vi "Init Wrist.vi"() -> (3 "Wrist Out":T2={"DeviceStatus"={"status"=FALSE, "code"=0, "source"=""}, "Type"=enum."CAN", "PWM"={"PWM Channel"=enum."PWM 1", "DeadBand"={"Name"="", "maxPositivePwm"=0, "minPositivePwm"=0, "centerPwm"=0, "maxNegativePwm"=0, "minNegativePwm"=0, "angularRange"=0}}, "CAN"={"Device Number"=1, "SetOutput VI Ref"=variant(refnum<vi> refnum), "GetOutput VI Ref"=variant(refnum<vi> refnum), "Enable VI Ref"=variant(refnum<vi> refnum), "Disable VI Ref"=variant(refnum<vi> refnum), "Data"=variant(cluster{"Library":path, "handle":u64, "Control Mode":u16, "UsageFrame":u32, "RefNumName":string, "arbID":u32} {"Library"=path "libCTRE_PhoenixCCI.so", "handle"=2992853744, "Control Mode"=0, "UsageFrame"=0, "RefNumName"="Wrist", "arbID"=33816577})}, "Invert"=FALSE, "DIO PWM"={"PWM \"Enable\" Channel"=enum."Invalid", "DIOChannel"=enum."Invalid", "PWM Rate"=0.0}})   [LabVIEW 2018]
uses:
  <vilib>/Rock Robotics/WPI/MotorControl/WPI_MotorControlDeviceRef.ctl
  <vilib>/Rock Robotics/WPI/MotorControl/WPI_MotorControlType.ctl
  <vilib>/Rock Robotics/SystemInterfaces/DIO/FPGA_DIOPWMChannel.ctl
  <vilib>/Rock Robotics/WPI/PWM/WPI_PWMDeadband.ctl
  <vilib>/Rock Robotics/SystemInterfaces/DIO/FPGA_DIOChannel.ctl
  <vilib>/Rock Robotics/WPI/ThirdParty/Phoenix-LabVIEW/Motor Controller/Controls/CTRE_Phoenix_MotorControl_NeutralMode.ctl
  <vilib>/Rock Robotics/WPI/ThirdParty/Phoenix-LabVIEW/Motor Controller/Controls/CTRE_Phoenix_MotorControl_FeedbackDevice.ctl
panel:
  in  "Deadband":dbl
  in  "Max Velocity":i32=1000
  in  "Max Accel":i32=1000
  in  "PID Constants":T1={"P Gain"=1.0, "I Gain"=0.002, "D Gain"=0.1, "F Gain"=0.0, "I Zone"=300.0, "Min Output"=-1.0, "Max Output"=1.0}
  in  "Enable Current Limit?":bool=TRUE
  in  "Peak Current Maximum Duration (ms)":i32
  in  "Peak Current (Amps)":i32
  in  "Continuous Current Limit (Amps)":i32=30
  in  "Invert":bool=TRUE
  in  "Sensor Inverted":bool=TRUE
  in  "Device Number":u8=5
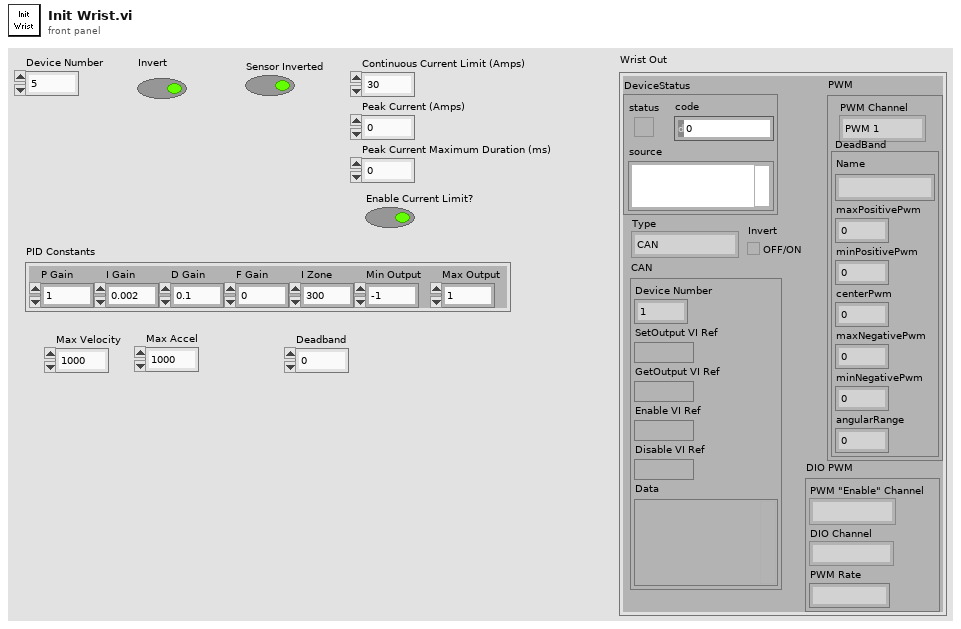
[diagram p1: front panel]
types:
  T1 = cluster{"P Gain":dbl, "I Gain":dbl, "D Gain":dbl, "F Gain":dbl, "I Zone":dbl, "Min Output":dbl, "Max Output":dbl}
  T2 = typedef "WPI_MotorControlDeviceRef.ctl" = cluster{"DeviceStatus":errorcluster, "Type":T3, "PWM":cluster{"PWM Channel":T4, "DeadBand":T5}, "CAN":cluster{"Device Number":u8, "SetOutput VI Ref":variant, "GetOutput VI Ref":variant, "Enable VI Ref":variant, "Disable VI Ref":variant, "Data":variant}, "Invert":bool, "DIO PWM":cluster{"PWM \"Enable\" Channel":T4, "DIOChannel":T6, "PWM Rate":dbl}}
  T3 = typedef "WPI_MotorControlType.ctl" = enum16{"PWM", "CAN", "DIO PWM"}
  T4 = typedef "FPGA_DIOPWMChannel.ctl" = enum8{"PWM 0", "PWM 1", "PWM 2", "PWM 3", "PWM 4", "PWM 5", "PWM 6", "PWM 7", "PWM 8", "PWM 9", "PWM MXP 0", "PWM MXP 1", "PWM MXP 2", "PWM MXP 3", "PWM MXP 4", "PWM MXP 5", "PWM MXP 6", "PWM MXP 7", "PWM MXP 8", "PWM MXP 9", "Invalid"}
  T5 = typedef "WPI_PWMDeadband.ctl" = cluster{"Name":string, "maxPositivePwm":i32, "minPositivePwm":i32, "centerPwm":i32, "maxNegativePwm":i32, "minNegativePwm":i32, "angularRange":u16}
  T6 = typedef "FPGA_DIOChannel.ctl" = enum8{"DIO 0", "DIO 1", "DIO 2", "DIO 3", "DIO 4", "DIO 5", "DIO 6", "DIO 7", "DIO 8", "DIO 9", "DIO MXP 0", "DIO MXP 1", "DIO MXP 2", "DIO MXP 3", "DIO MXP 4", "DIO MXP 5", "DIO MXP 6", "DIO MXP 7", "DIO MXP 8", "DIO MXP 9", "DIO MXP 10", "DIO MXP 11", "DIO MXP 12", "DIO MXP 13", "DIO MXP 14", "DIO MXP 15", "SPI Port CS1", "SPI Port CS2", "SPI Port CS3", "SPI Port MISO", "SPI Port MOSI", "Invalid"}
  T7 = typedef "CTRE_Phoenix_MotorControl_FeedbackDevice.ctl" = i8
  T8 = typedef "CTRE_Phoenix_MotorControl_NeutralMode.ctl" = enum8{"EEPROMSetting", "Override to Coast", "Override to Brake"}
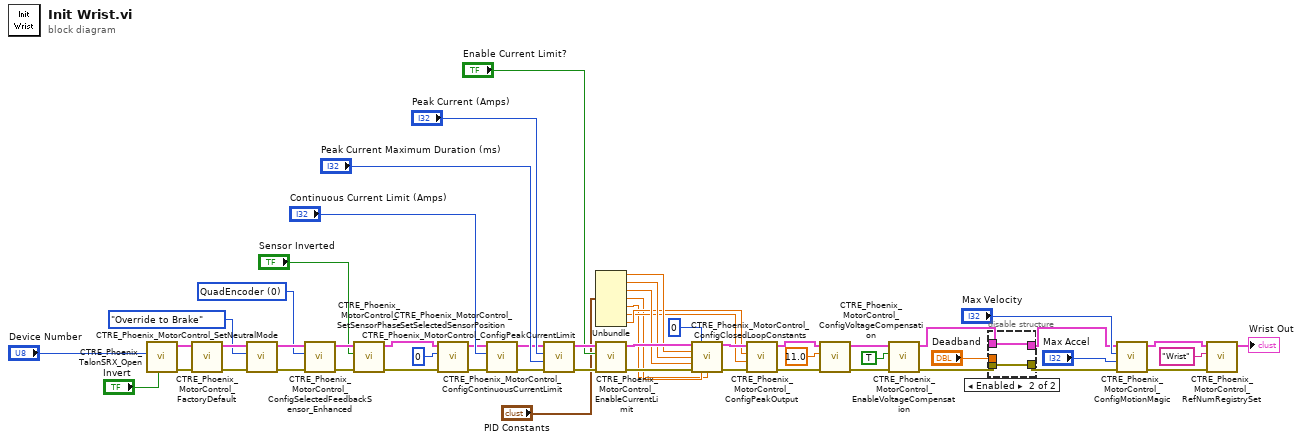
[diagram p0: block diagram]
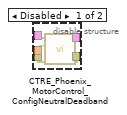
[diagram p2: hidden frame]
diagram:
  w47 = T7 0 items=["QuadEncoder"=0, "Analog"=2, "Tachometer"=4, "Pulse Width Encoded Position"=8, "Sensor Sum (S0 + S1)"=9, "Sensor Difference (D0 - D1)"=10, "Remote Source 0"=11, "Remote Source 1"=12, "Software Emulated"=15] ("Feedback Device")
  n1 = call <vilib>:"CTRE_Phoenix_TalonSRX_Open.vi"("Invert"="Invert", "Device Number"="Device Number") -> ("error out"=w54:errorcluster, "CAN Talon SRX Ref"=w53:T2)  [unwired: 8 in]
  n2 = call <vilib>:"CTRE_Phoenix_MotorControl_FactoryDefault.vi"("error in"=w54, "PhoenixMotorControlDevRef"=w53) -> ("error out"=w51:errorcluster, "PhoenixMotorControlDevRef"=w52:T2)  [unwired: 8 in]
  n3 = call <vilib>:"CTRE_Phoenix_MotorControl_SetNeutralMode.vi"("error in (no error)"=w51, "Motor Control Neutral Mode"=CTRE_Phoenix_MotorControl_NeutralMode."Override to Brake", "PhoenixMotorControlDevRef"=w52) -> ("error out"=w48:errorcluster, "PhoenixMotorControlDevRef"=w49:T2)  [unwired: 7 in]
  n4 = call <vilib>:"CTRE_Phoenix_MotorControl_ConfigSelectedFeedbackSensor_Enhanced.vi"("error in (no error)"=w48, "Feedback Device"=w47, "PhoenixMotorControlDevRef"=w49) -> ("error out"=w45:errorcluster, "PhoenixMotorControlDevRef"=w46:T2)  [unwired: 7 in]
  n5 = call <vilib>:"CTRE_Phoenix_MotorControl_SetSensorPhase.vi"("error in (no error)"=w45, "PhaseSensor"="Sensor Inverted", "PhoenixMotorControlDevRef"=w46) -> ("error out"=w42:errorcluster, "PhoenixMotorControlDevRef"=w43:T2)  [unwired: 7 in]
  n6 = call <vilib>:"CTRE_Phoenix_MotorControl_SetSelectedSensorPosition.vi"("error in (no error)"=w42, "New Sensor Position"=0, "PhoenixMotorControlDevRef"=w43) -> ("error out"=w32:errorcluster, "PhoenixMotorControlDevRef"=w33:T2)  [unwired: 7 in]
  n7 = call <vilib>:"CTRE_Phoenix_MotorControl_ConfigContinuousCurrentLimit.vi"("error in (no error)"=w32, "Continuous Current Limit (Amps)"="Continuous Current Limit (Amps)", "PhoenixMotorControlDevRef"=w33) -> ("error out"=w36:errorcluster, "PhoenixMotorControlDevRef"=w37:T2)  [unwired: 7 in]
  n8 = call <vilib>:"CTRE_Phoenix_MotorControl_ConfigPeakCurrentLimit.vi"("error in (no error)"=w36, "Peak Current Maximum Duration (ms)"="Peak Current Maximum Duration (ms)", "Peak Current (Amps)"="Peak Current (Amps)", "PhoenixMotorControlDevRef"=w37) -> ("error out"=w34:errorcluster, "PhoenixMotorControlDevRef"=w35:T2)  [unwired: 6 in]
  n9 = Unbundle("PID Constants") -> ("P Gain"=w26:dbl, "I Gain"=w25:dbl, "D Gain"=w24:dbl, "F Gain"=w19:dbl, "I Zone"=w18:dbl, "Min Output"=w20:dbl, "Max Output"=w21:dbl)
  n10 = call <vilib>:"CTRE_Phoenix_MotorControl_EnableCurrentLimit.vi"("error in (no error)"=w34, "Enable Current Limit?"="Enable Current Limit?", "PhoenixMotorControlDevRef"=w35) -> ("error out"=w27:errorcluster, "PhoenixMotorControlDevRef"=w28:T2)  [unwired: 7 in]
  n11 = call <vilib>:"CTRE_Phoenix_MotorControl_ConfigClosedLoopConstants.vi"("PhoenixMotorControlDevRef"=w28, "slotIdx"=0, "P"=w26, "I"=w25, "D"=w24, "error in (no error)"=w27, "F"=w19, "I Zone"=w18) -> ("PhoenixMotorControlDevRef"=w22:T2, "error out"=w23:errorcluster)  [unwired: 6 in]
  n12 = call <vilib>:"CTRE_Phoenix_MotorControl_ConfigPeakOutput.vi"("error in (no error)"=w23, "Reverse Peak Percent Output"=w20, "Forward Peak Percent Output"=w21, "PhoenixMotorControlDevRef"=w22) -> ("error out"=w9:errorcluster, "PhoenixMotorControlDevRef"=w10:T2)  [unwired: 6 in]
  n13 = call <vilib>:"CTRE_Phoenix_MotorControl_ConfigVoltageCompensation.vi"("error in (no error)"=w9, "Saturation Voltage"=11.0, "PhoenixMotorControlDevRef"=w10) -> ("error out"=w8:errorcluster, "PhoenixMotorControlDevRef"=w7:T2)  [unwired: 7 in]
  n14 = call <vilib>:"CTRE_Phoenix_MotorControl_EnableVoltageCompensation.vi"("error in (no error)"=w8, "Enable Voltage Compensation?"=TRUE, "PhoenixMotorControlDevRef"=w7) -> ("error out"=w2:errorcluster, "PhoenixMotorControlDevRef"=w5:T2)  [unwired: 7 in]
  n15 = disable-structure shown="Enabled" {
    disable-tunnel: w5 -> [w61 w63]
    disable-tunnel: [w60 w63] -> w4
    disable-tunnel: [w59 w62] -> w3
    disable-tunnel: w2 -> [w58 w62]
    disable-tunnel: "Deadband" -> [w57 _]
    frame Disabled {
      n16 = call <vilib>:"CTRE_Phoenix_MotorControl_ConfigNeutralDeadband.vi"("error in (no error)"=w58, "Percent Deadband"=w57, "PhoenixMotorControlDevRef"=w61) -> ("error out"=w59:errorcluster, "PhoenixMotorControlDevRef"=w60:T2)  [unwired: 7 in]
    }
    frame Enabled {
    }
  }
  n17 = call <vilib>:"CTRE_Phoenix_MotorControl_ConfigMotionMagic.vi"("error in (no error)"=w3, "Acceleration"="Max Accel", "Cruise Velocity"="Max Velocity", "PhoenixMotorControlDevRef"=w4) -> ("error out"=w13:errorcluster, "PhoenixMotorControlDevRef"=w14:T2)  [unwired: 6 in]
  n18 = call <vilib>:"CTRE_Phoenix_MotorControl_RefNumRegistrySet.vi"("error in (no error)"=w13, "refnum name"="Wrist", "PhoenixMotorControlDevRef"=w14) -> ("PhoenixMotorControlDevRef"=→"Wrist Out":T2)  [unwired: 7 in, 1 out]
